vi "Init.vi"(7 "EDS":refnum<class "Electronic Datasheet.lvclass">, 8 "error in":errorcluster, 10 "OD Entry":refnum<class "OD Entry.lvclass">, 11 "TPDO Mapping in":refnum<class "TX PDO Mapping.lvclass">) -> (0 "error out":errorcluster, 3 "TPDO Mapping out":refnum<class "TX PDO Mapping.lvclass">)   [LabVIEW 2024, in "PDO Grid.lvlib" / "TX PDO Mapping.lvclass"]
uses:
  TX PDO Mapping.lvclass
  TX PDO Mapping.lvclass/TX PDO Mapping.ctl
  Core/OD Entry/OD Entry.lvclass
  Core/Value/Value.lvclass
  PDO Mapping/PDO Mapping.lvclass
  Core/OD Sub-Entry/OD Sub-Entry.lvclass
  D:/git/EDS-File-Viewer/Core/OD Entry/OD Entry.lvclass
  D:/git/EDS-File-Viewer/Core/OD Sub-Entry/OD Sub-Entry.lvclass
  Electronic Datasheet/Electronic Datasheet.lvclass
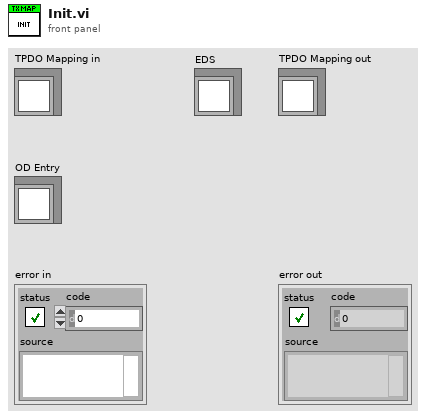
[diagram p1: front panel]
types:
  T1 = typedef "Electronic Datasheet.lvlib/Access Type.ctl" = enum16{"ro", "wo", "rw", "rwr", "rww", "const"}
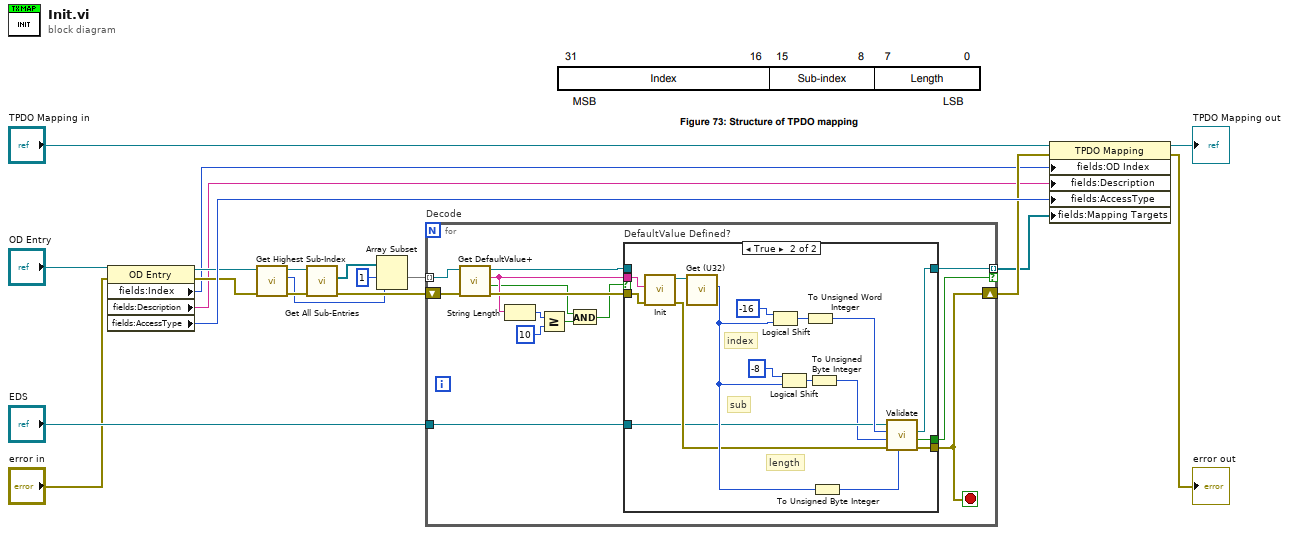
[diagram p0: block diagram]
diagram:
  n1 = property class="OD Entry"(reference="OD Entry", error in="error in") -> (reference out=w9:refnum<class "OD Entry.lvclass">, error out=w7:errorcluster, "fields:Index"=w4:u16, "fields:Description"=w5:string, "fields:AccessType"=w18:T1)
  n2 = call "Get Highest Sub-Index.vi"("Error In"=w7, "reference in"=w9) -> ("Error Out"=w10:errorcluster, "Highes Sub-Index"=w6:i16, "reference out"=w8:refnum<class "OD Entry.lvclass">)  [unwired: 7 in]
  n3 = call "Get All Sub-Entries.vi"("Error In"=w10, "reference in"=w8) -> ("Error Out"=w14:errorcluster, "Sub-Entries"=w12:refnum<class "OD Sub-Entry.lvclass">[])  [unwired: 6 in, 2 out]
  n4 = Array Subset(array=w12, index=1, length=w6) -> (w13:refnum<class "OD Sub-Entry.lvclass">[])
  n5 = for "Decode" {
    tunnel: "EDS" -> [w31]
    shift-right: [w28] -> w16
    shift-left: w14 -> [w34]
    tunnel: [w30] -> w3 mode=indexing if=w29
    tunnel: w13 -> [w27] mode=indexing
    stop <- w28 stop-if-true
    n6 = call "Get DefaultValue+.vi"("Error In"=w34, "reference in"=w27) -> ("Error Out"=w32:errorcluster, "Defined?"=w22:bool, "DefaultValue"=w26:string, "reference out"=w33:refnum<class "OD Sub-Entry.lvclass">)  [unwired: 6 in]
    n7 = String Length(string=w26) -> (length=w25:i32)
    n8 = Greater Or Equal?(x=w25, y=10) -> (x >= y?=w23:bool)
    n9 = And(x=w22, y=w23) -> (x .and. y?=w21:bool)
    n10 = case "DefaultValue Defined?" shown="True" w21 {
      selector: w21 -> [w35 _]
      tunnel: w33 -> [w36 _]
      tunnel: w26 -> [_ w52]
      tunnel: w32 -> [w37 w53]
      tunnel: w31 -> [_ w45]
      tunnel: [w37 w44] -> w28
      tunnel: [w36 w38] -> w30
      tunnel: [w35 w39] -> w29
      frame False {
      }
      frame True {
        # "length"
        # "index"
        # "sub"
        n11 = call "Init.vi"("error in"=w53, "Value"=w52) -> ("error out"=w46:errorcluster, "Value out"=w51:refnum<class "Value.lvclass">)  [unwired: 8 in]
        n12 = call "Get (U32).vi"("Value in"=w51) -> ("Value"=w49:u32)  [unwired: 8 in, 2 out]
        n13 = Logical Shift(y=i16 -16, x=w49) -> (x << y=w43:u32)
        n14 = Logical Shift(y=i16 -8, x=w49) -> (x << y=w42:u32)
        n15 = To Unsigned Word Integer(number=w43) -> (unsigned 16bit integer=w47:u16)
        n16 = To Unsigned Byte Integer(number=w42) -> (unsigned 8bit integer=w41:u8)
        n17 = To Unsigned Byte Integer(number=w49) -> (unsigned 8bit integer=w40:u8)
        n18 = call "Validate.vi"("Length"=w40, "error in"=w46, "Sub-Index"=w41, "Index"=w47, "EDS"=w45) -> ("error out"=w44:errorcluster, "Valid?"=w39:bool, "Mapping Target"=w38:refnum<class "OD Entry.lvclass">)  [unwired: 4 in]
      }
    }
  }
  n19 = property class="TPDO Mapping"(reference="TPDO Mapping in", error in=w16, "fields:OD Index"=w4, "fields:Description"=w5, "fields:AccessType"=w18, "fields:Mapping Targets"=w3) -> (reference out=→"TPDO Mapping out":refnum<class "TX PDO Mapping.lvclass">, error out=→"error out":errorcluster)
